vi "Test RaspberryPiPico API.vi"() -> ()   [LabVIEW 2020]
doc: "RaspberryPiPico API Tester."
uses:
  <instrlib>/HandsOnPi2040/cti-drivers-lv-visa-main/CTI-Visa/Identity.ctl
  <vilib>/Utility/error.llb/DialogType.ctl
  RaspberryPiPico.lvlib
  <instrlib>/HandsOnPi2040/cti-drivers-lv-visa-main/CTI-Visa/CTI-Visa.lvlib
panel:
  out "Map":map{i32, bool[]}(c390)
  out "Analog Inputs":u16[](graph)
  out "Instrument Connection Status":bool
  in  "Initialize Instrument":bool
  out "Identity":T1
  in  "VISA resource name":refnum<visa-resource-name>="TCPIP0::192.168.0.171::6340::SOCKET"
  out "last error":errorcluster
  in  "Show Diagram on Init":bool
  in  "Run as Singleton?":bool
  in  "Show Block Diagram":bool
  in  "Refresh Modules":bool
  out "Active Modules":string[](array[string])
  in  "Stop Module":bool
  in  "Select Module":i32(ring)=-1 caption="Select Module\nTo send Request to" items=["All"=-1, "2"=2]
  in  "Run New Module":bool
  in  "Hide Module Panel":bool
  in  "Show Module Panel":bool
  out "Status":string
  # "This VI tests the API for the Module."
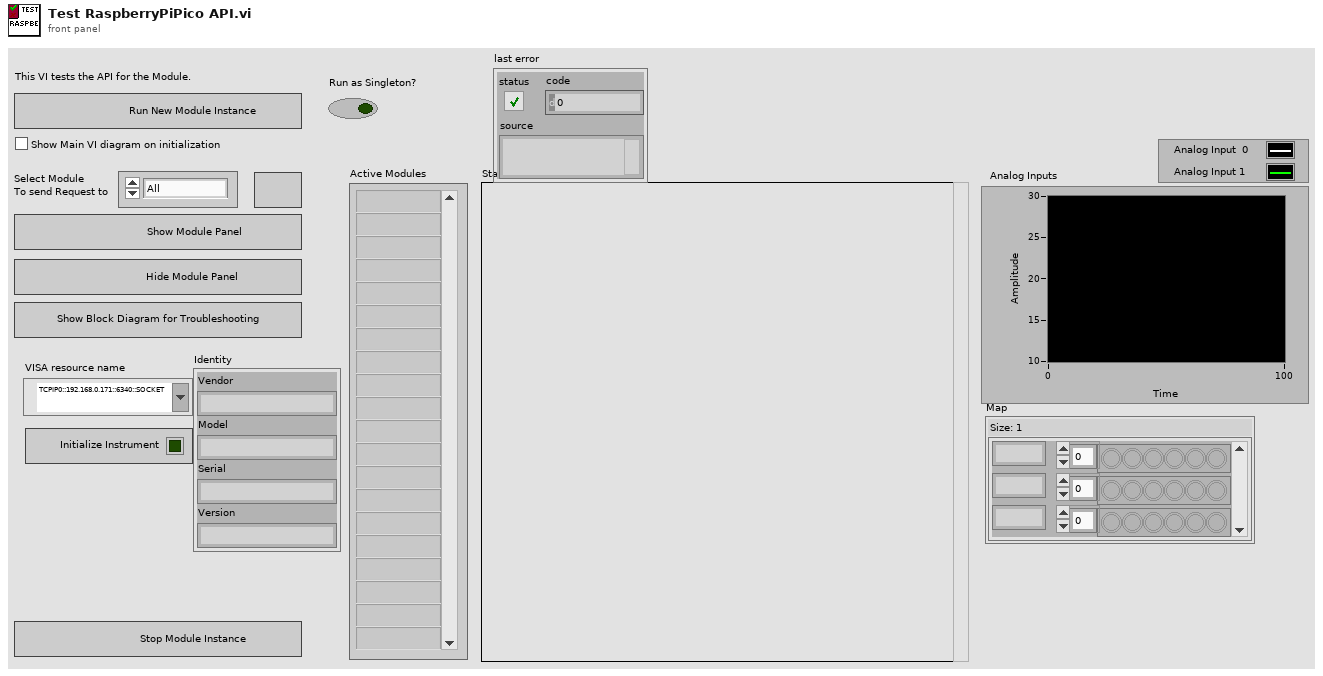
[diagram p1: front panel]
types:
  T1 = typedef "CTI-Visa.lvlib/Identity.ctl" = cluster{"Vendor":string, "Model":string, "Serial":string, "Version":string}
  T2 = typedef "RaspberryPiPico.lvlib/Broadcast Events--cluster.ctl" = cluster{"Module Did Init":refnum<user-event>, "Status Updated":refnum<user-event>, "Error Reported":refnum<user-event>, "Module Did Stop":refnum<user-event>, "Update Module Execution Status":refnum<user-event>, "Instrument Connected":refnum<user-event>, "Analog Inputs Updated":refnum<user-event>, "Digital Inputs Updated":refnum<user-event>}
  T3 = typedef "DialogType.ctl" = u16
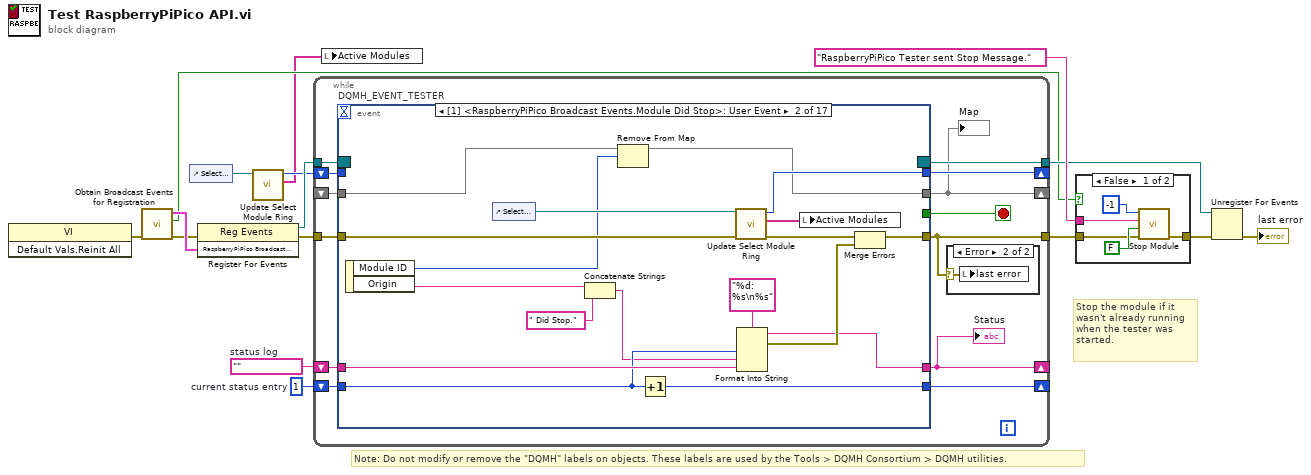
[diagram p0: block diagram]
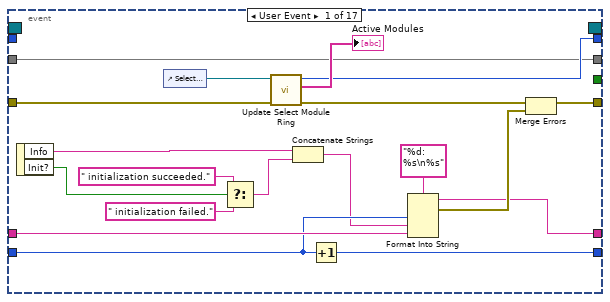
[diagram p4: hidden frame]
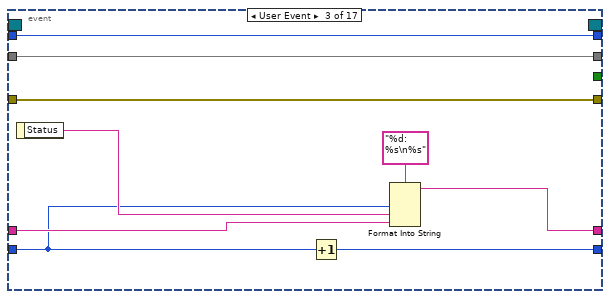
[diagram p5: hidden frame]
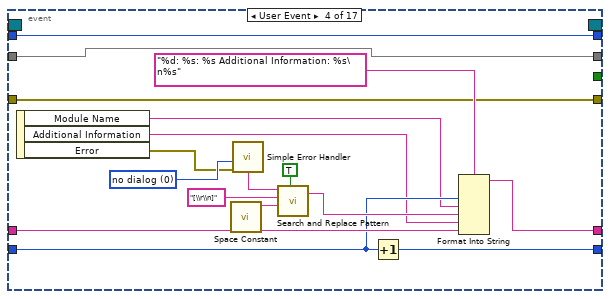
[diagram p6: hidden frame]
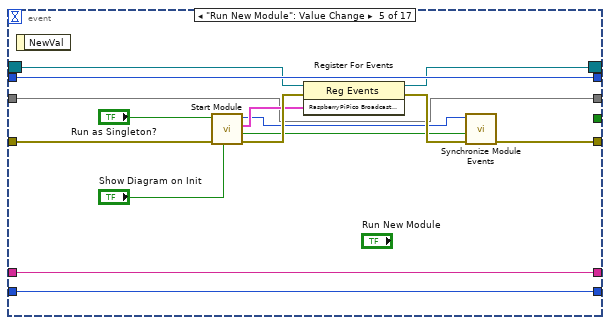
[diagram p7: hidden frame]
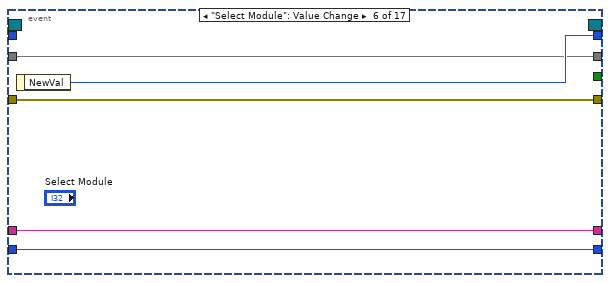
[diagram p8: hidden frame]
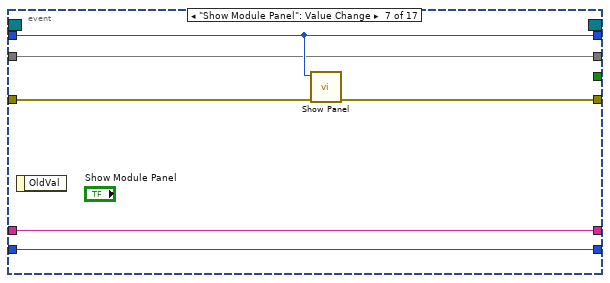
[diagram p9: hidden frame]
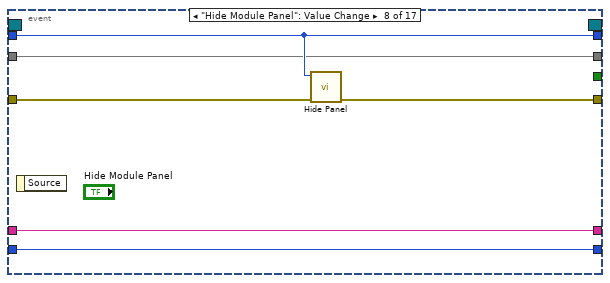
[diagram p10: hidden frame]
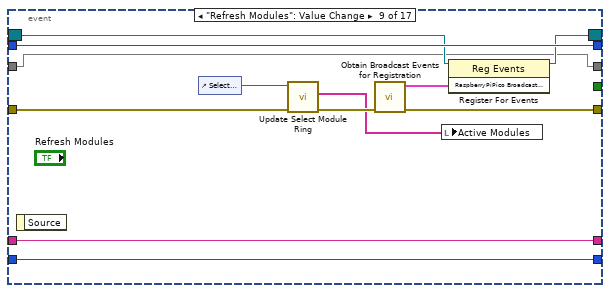
[diagram p11: hidden frame]
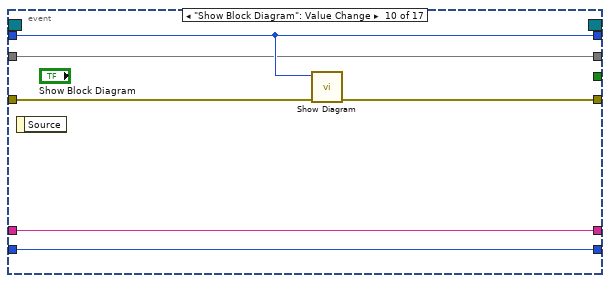
[diagram p12: hidden frame]
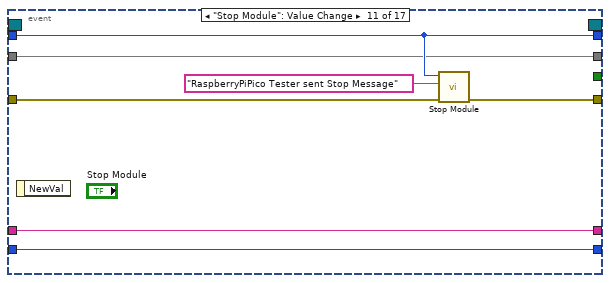
[diagram p13: hidden frame]
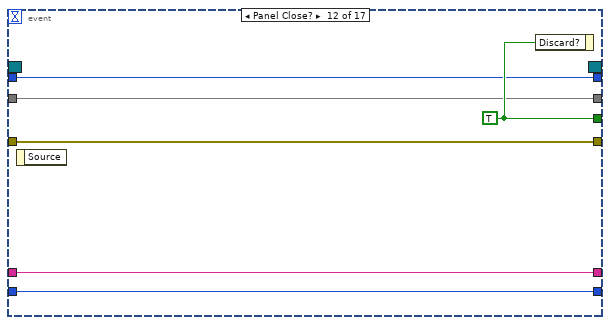
[diagram p14: hidden frame]
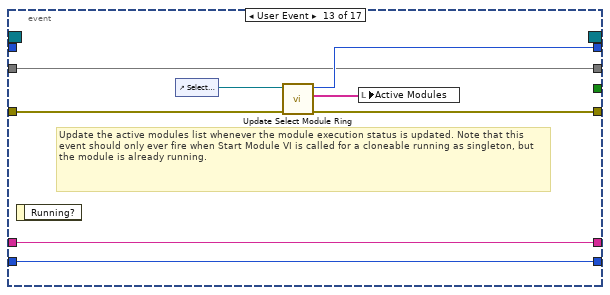
[diagram p15: hidden frame]
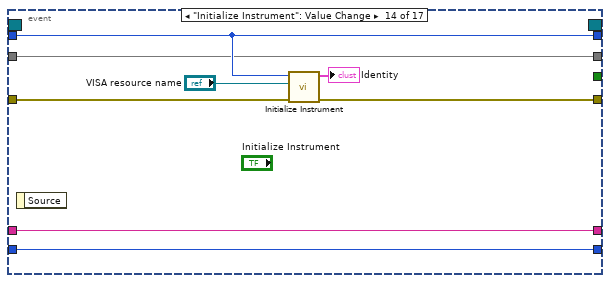
[diagram p16: hidden frame]
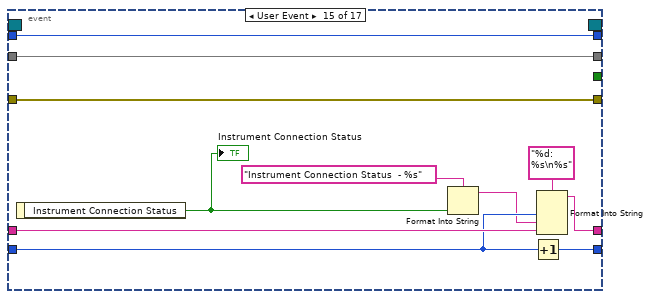
[diagram p17: hidden frame]
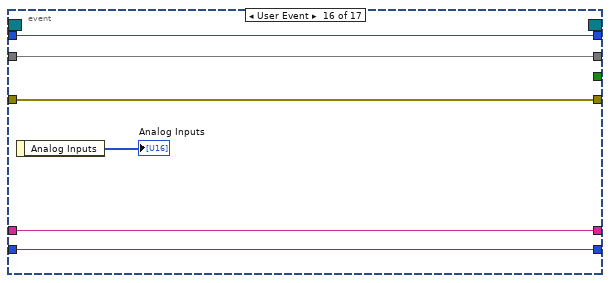
[diagram p18: hidden frame]
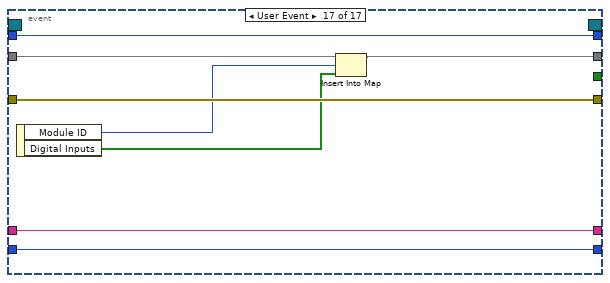
[diagram p19: hidden frame]
diagram:
  w13 = 1  # current status entry
  w14 = ""  # status log
  # "Stop the module if it wasn't already running when the tester was started."
  # "Note: Do not modify or remove the \"DQMH\" labels on objects. These labels are used by the Tools > DQMH Consortium > DQMH utilities."
  n1 = invoke class="VI" method="Default Vals.Reinit All"() -> (error out=w8:errorcluster)  [unwired: 3 in, 2 out]
  n2 = call "Obtain Broadcast Events for Registration.vi"("error in"=w8) -> ("error out"=w7:errorcluster, "Already running?"=w6:bool, "RaspberryPiPico Broadcast Events"=w12:T2)  [unwired: 8 in]
  n3 = control-ref of="Select Module"() -> (w3:refnum<vi>)
  n4 = register-events(error in=w7, w12) -> (reference out=w16:refnum<event-registration>, error out=w11:errorcluster)  [unwired: 1 in]
  n5 = call "Update Select Module Ring.vi"("Select Module Ring Ref"=w3) -> ("Active Modules (Array)"=w1:string[], "New Module Ring Value"=w2:i32)  [unwired: 8 in, 1 out]
  n6 = while {
    tunnel: w16 -> [w29]
    tunnel: [w20] -> w5
    tunnel: w11 -> [w28]
    shift-right: [w24] -> _
    shift-left: w14 -> [w26]
    shift-right: [w25] -> _
    shift-left: w13 -> [w27]
    shift-right: [w22] -> _
    shift-left: w2 -> [w23]
    tunnel: [w21] -> w9
    shift-right: [w18] -> _
    shift-left: _ -> [w17]
    stop <- w19 stop-if-true
    n7 = event "DQMH_EVENT_TESTER" shown="[1] <RaspberryPiPico Broadcast Events.Module Did Stop>: User Event" {
      selector: w29 -> [_ _ _ _ w102 _ _ _ w132 _ _ _ _ _ _ _ _]
      dyn-events: [_ _ _ _ w101 _ _ _ w131 _ _ _ _ _ _ _ _] -> w21
      timeout: _ -> [_ _ _ _ _ _ _ _ _ _ _ _ _ _ _ _ _]
      tunnel: [_ _ _ _ _ _ _ _ _ _ _ w156 _ _ _ _ _] -> w19
      tunnel: [w39 w59 w76 w81 w100 w113 w118 w124 w128 w140 w146 w155 w160 w168 w183 w189 w197] -> w20
      tunnel: w28 -> [w41 w61 w76 w81 w103 w113 w119 w125 w133 w143 w147 w155 w161 w172 w183 w189 w197]
      tunnel: w27 -> [w46 w64 w69 w84 w105 w111 w116 w122 w136 w141 w149 w153 w163 w170 w179 w186 w194]
      tunnel: w26 -> [w47 w65 w72 w85 w106 w112 w117 w123 w137 w142 w150 w154 w164 w171 w181 w187 w195]
      tunnel: [w44 w62 w73 w83 w106 w112 w117 w123 w137 w142 w150 w154 w164 w171 w180 w187 w195] -> w24
      tunnel: [w45 w63 w75 w82 w105 w111 w116 w122 w136 w141 w149 w153 w163 w170 w178 w186 w194] -> w25
      tunnel: w23 -> [_ _ w70 w93 w104 _ w115 w121 w135 w139 w148 w152 _ w169 w182 w188 w196]
      tunnel: [w36 w56 w70 w93 w104 w110 w115 w121 w135 w139 w148 w152 w159 w169 w182 w188 w196] -> w22
      tunnel: [w31 w51 w68 w77 w94 w109 w114 w120 w126 w138 w144 w151 w157 w165 w173 w184 w191] -> w18
      tunnel: w17 -> [w31 w52 w68 w77 w94 w109 w114 w120 w126 w138 w144 w151 w157 w165 w173 w184 w190]
      event User Event {
        n8 = event-data() -> ("Info"=w43:string, "Init?"=w33:bool)  [unwired: 1 in]
        n9 = control-ref of="Select Module"() -> (w38:refnum<vi>)
        n10 = Select(t=" initialization succeeded.", s=w33, f=" initialization failed.") -> (s? t:f=w32:string)
        n11 = call "Update Select Module Ring.vi"("error in"=w41, "Select Module Ring Ref"=w38) -> ("error out"=w40:errorcluster, "Active Modules (Array)"=→"Active Modules":string[], "New Module Ring Value"=w36:i32)  [unwired: 7 in]
        n12 = Concatenate Strings(w43, w32) -> (w42:string)
        n13 = Increment(x=w46) -> (x+1=w45:i32)
        n14 = Format Into String(format string="%d: %s\n%s", w46, w42, w47) -> (resulting string=w44:string, error out=w49:errorcluster)  [unwired: 2 in]
        n15 = Merge Errors(w40, w49) -> (w39:errorcluster)
      }
      event User Event {
        n16 = event-data() -> ("Module ID"=w50:i32, "Origin"=w54:string)  [unwired: 1 in]
        n17 = control-ref of="Select Module"() -> (w58:refnum<vi>)
        n18 = Concatenate Strings(w54, " Did Stop.") -> (w53:string)
        n19 = Remove From Map(10:w50, 11:w52) -> (3:w51:map{i32, bool[]})  [unwired: 2 out]
        n20 = Increment(x=w64) -> (x+1=w63:i32)
        n21 = call "Update Select Module Ring.vi"("error in"=w61, "Select Module Ring Ref"=w58) -> ("error out"=w60:errorcluster, "Active Modules (Array)"=w57:string[], "New Module Ring Value"=w56:i32)  [unwired: 7 in]
        n22 = Format Into String(format string="%d: %s\n%s", w64, w53, w65) -> (resulting string=w62:string, error out=w67:errorcluster)  [unwired: 2 in]
        n23 = local write "Active Modules"(w57) -> ()
        n24 = Merge Errors(w60, w67) -> (w59:errorcluster)
      }
      event User Event {
        n25 = event-data() -> ("Status"=w71:string)  [unwired: 1 in]
        n26 = Increment(x=w69) -> (x+1=w75:i32)
        n27 = Format Into String(format string="%d: %s\n%s", w69, w71, w72) -> (resulting string=w73:string)  [unwired: 2 in, 1 out]
      }
      event User Event {
        w86 = T3 0 items=["no dialog", "OK message", "continue or stop message", "OK message + warnings", "continue/stop + warnings"] ("type of dialog (OK msg:1)")
        n28 = event-data() -> ("Module Name"=w80:string, "Additional Information"=w79:string, "Error"=w78:errorcluster)  [unwired: 1 in]
        n29 = call <vilib>:"Space Constant.vi"() -> ("String"=w90:string)
        n30 = call <vilib>:"Simple Error Handler.vi"("type of dialog (OK msg:1)"=w86, "error in (no error)"=w78) -> ("message"=w87:string)  [unwired: 3 in, 4 out]
        n31 = call <vilib>:"Search and Replace Pattern.vi"("string"=w87, "regular expression (\"\")"="[\\r\\n]" ("regular expression (\"\")"), "replace string (\"\")"=w90, "replace all? (F)"=TRUE ("replace all CR/LF with spaces")) -> ("result string"=w88:string)  [unwired: 1 in, 1 out]
        n32 = Increment(x=w84) -> (x+1=w82:i32)
        n33 = Format Into String(format string="%d: %s: %s Additional Information: %s\n%s", w84, w80, w88, w79, w85) -> (resulting string=w83:string)  [unwired: 2 in, 1 out]
      }
      event "Run New Module": Value Change {
        n34 = event-data() -> ()  [unwired: 1 in, 1 out]
        n35 = call "Start Module.vi"("Show Main VI Diagram on Init (F)"="Show Diagram on Init", "error in"=w103, "Run as Singleton? (F)"="Run as Singleton?") -> ("error out"=w107:errorcluster, "Wait for Event Sync?"=w99:bool, "RaspberryPiPico Broadcast Events"=w98:T2, "Module ID"=w95:i32)  [unwired: 4 in, 1 out]
        n36 = register-events(reference=w102, error in=w107, w98) -> (reference out=w101:refnum<event-registration>, error out=w108:errorcluster)
        n37 = call "Synchronize Module Events.vi"("error in"=w108, "Wait for Event Sync?"=w99, "Module ID in"=w95) -> ("error out"=w100:errorcluster)  [unwired: 7 in, 1 out]
      }
      event "Select Module": Value Change {
        n38 = event-data() -> ("NewVal"=w110:i32)  [unwired: 1 in]
      }
      event "Show Module Panel": Value Change {
        n39 = event-data() -> ()  [unwired: 1 in, 1 out]
        n40 = call "Show Panel.vi"("error in"=w119, "Module ID"=w115) -> ("error out"=w118:errorcluster)  [unwired: 9 in]
      }
      event "Hide Module Panel": Value Change {
        n41 = event-data() -> ()  [unwired: 1 in, 1 out]
        n42 = call "Hide Panel.vi"("error in"=w125, "Module ID"=w121) -> ("error out"=w124:errorcluster)  [unwired: 9 in]
      }
      event "Refresh Modules": Value Change {
        n43 = event-data() -> ()  [unwired: 1 in, 1 out]
        n44 = control-ref of="Select Module"() -> (w134:refnum<vi>)
        n45 = call "Update Select Module Ring.vi"("error in"=w133, "Select Module Ring Ref"=w134) -> ("error out"=w129:errorcluster, "Active Modules (Array)"=w127:string[])  [unwired: 7 in, 1 out]
        n46 = call "Obtain Broadcast Events for Registration.vi"("error in"=w129) -> ("error out"=w128:errorcluster, "RaspberryPiPico Broadcast Events"=w130:T2)  [unwired: 8 in, 1 out]
        n47 = local write "Active Modules"(w127) -> ()
        n48 = register-events(reference=w132, w130) -> (reference out=w131:refnum<event-registration>)  [unwired: 1 in, 1 out]
      }
      event "Show Block Diagram": Value Change {
        n49 = event-data() -> ()  [unwired: 1 in, 1 out]
        n50 = call "Show Diagram.vi"("error in"=w143, "Module ID"=w139) -> ("error out"=w140:errorcluster)  [unwired: 9 in]
      }
      event "Stop Module": Value Change {
        n51 = event-data() -> ()  [unwired: 1 in, 1 out]
        n52 = call "Stop Module.vi"("error in"=w147, "Origin"="RaspberryPiPico Tester sent Stop Message", "Module ID"=w148) -> ("error out"=w146:errorcluster)  [unwired: 8 in]
      }
      event Panel Close? {
        w156 = TRUE ("Discard?")
        n53 = event-data() -> ()  [unwired: 1 in, 1 out]
        n54 = event-data("Discard?"=w156) -> ()  [unwired: 1 in, 1 out]
      }
      event User Event {
        # "Update the active modules list whenever the module execution status is updated. Note that this event should only ever fire when Start Module VI is called for a cloneable running as singleton, but the module is already running."
        n55 = event-data() -> ()  [unwired: 1 in, 1 out]
        n56 = control-ref of="Select Module"() -> (w162:refnum<vi>)
        n57 = call "Update Select Module Ring.vi"("error in"=w161, "Select Module Ring Ref"=w162) -> ("error out"=w160:errorcluster, "Active Modules (Array)"=w158:string[], "New Module Ring Value"=w159:i32)  [unwired: 7 in]
        n58 = local write "Active Modules"(w158) -> ()
      }
      event "Initialize Instrument": Value Change {
        n59 = event-data() -> ()  [unwired: 1 in, 1 out]
        n60 = call "Initialize Instrument.vi"("error in"=w172, "VISA resource name"="VISA resource name", "Module ID"=w169) -> ("error out"=w168:errorcluster, "Identity"=→"Identity":T1)  [unwired: 6 in, 1 out]
      }
      event User Event {
        n61 = event-data() -> ("Instrument Connection Status"=w174:bool)  [unwired: 1 in]
        "Instrument Connection Status" <- w174
        n62 = Format Into String(format string="Instrument Connection Status  - %s", w174) -> (resulting string=w175:string)  [unwired: 2 in, 1 out]
        n63 = Increment(x=w179) -> (x+1=w178:i32)
        n64 = Format Into String(format string="%d: %s\n%s", w179, w175, w181) -> (resulting string=w180:string)  [unwired: 2 in, 1 out]
      }
      event User Event {
        n65 = event-data() -> ("Analog Inputs"=→"Analog Inputs":u16[])  [unwired: 1 in]
      }
      event User Event {
        n66 = event-data() -> ("Module ID"=w193:i32, "Digital Inputs"=w192:bool[])  [unwired: 1 in]
        n67 = Insert Into Map(map in=w190, key=w193, value=w192) -> (map out=w191:map{i32, bool[]})  [unwired: 2 out]
      }
    }
    "Status" <- w24
    "Map" <- w18
    n68 = case shown="Error" w20 {
      selector: w20 -> [_ w30]
      frame No Error {
      }
      frame Error {
        n69 = local write "last error"(w30) -> ()
      }
    }
  }
  n70 = local write "Active Modules"(w1) -> ()
  n71 = case shown="False" w6 {
    tunnel: [w202 w203] -> w15
    tunnel: "RaspberryPiPico Tester sent Stop Message." ("Origin") -> [w201 _]
    tunnel: w5 -> [w198 w203]
    frame False {
      n72 = call "Stop Module.vi"("error in"=w198, "Wait for Module to stop? (F)"=FALSE ("Wait for Module to stop?"), "Origin"=w201, "Module ID"=-1 ("Stop all")) -> ("error out"=w202:errorcluster)  [unwired: 7 in]
    }
    frame True {
    }
  }
  n73 = Unregister For Events(event registration refnum=w9, error in=w15) -> (error out=→"last error":errorcluster)
